vi "ROI_boxes.vi"(11 "Camera Setup":T1={"Analog Gain (0-5)"=4, "Exposure Time"=0.01, "EM Gain (0-255)"=0, "Trigger Polarity"="ATP P", "External Trigger Mode"="ATP P", "Scan Speed"="EMD E", "External Trigger Source"="SSP H", "Scan Mode"="ESC B", "Super Pixel Binning\n(if enabled in Scan Mode)"="SMD N", "Camera Sub-array acquisition region\n(if enabled in scan mode)"={"Left"=0, "Top"=0, "Width"=0, "Height"=0}, "Use camera?"=FALSE, "# image buffers"=100, "shots per measurement"=100, "Force images to U16"=FALSE, "Low Light Sensitivity"="LLS 0", "cooling"="LLS 0", "fan"="LLS 0", "Frame Grabber acquisition region"={"Left"=0, "Top"=0, "Right"=0, "Bottom"=0}} {"Frame Grabber acquisition region"."Bottom" max=512 step=1; "Frame Grabber acquisition region"."Right" max=512 step=1; "Frame Grabber acquisition region"."Top" max=512 step=1; "Frame Grabber acquisition region"."Left" max=512 step=1; "shots per measurement" min=0 step=1; "# image buffers" min=0 step=1; "Camera Sub-array acquisition region\n(if enabled in scan mode)"."Height" min=16 max=512 step=16; "Camera Sub-array acquisition region\n(if enabled in scan mode)"."Width" min=16 max=512 step=16; "Camera Sub-array acquisition region\n(if enabled in scan mode)"."Top" max=496 step=16; "Camera Sub-array acquisition region\n(if enabled in scan mode)"."Left" max=496 step=16; "Analog Gain (0-5)" max=5 step=1}) -> (3 "ROI":T2)   [LabVIEW 2013]
uses:
  Camera/Hamamatsu_C9100-13/camera_setup.ctl
  Camera/Hamamatsu_C9100-13/Hamamatsu_C9100-13.lvclass
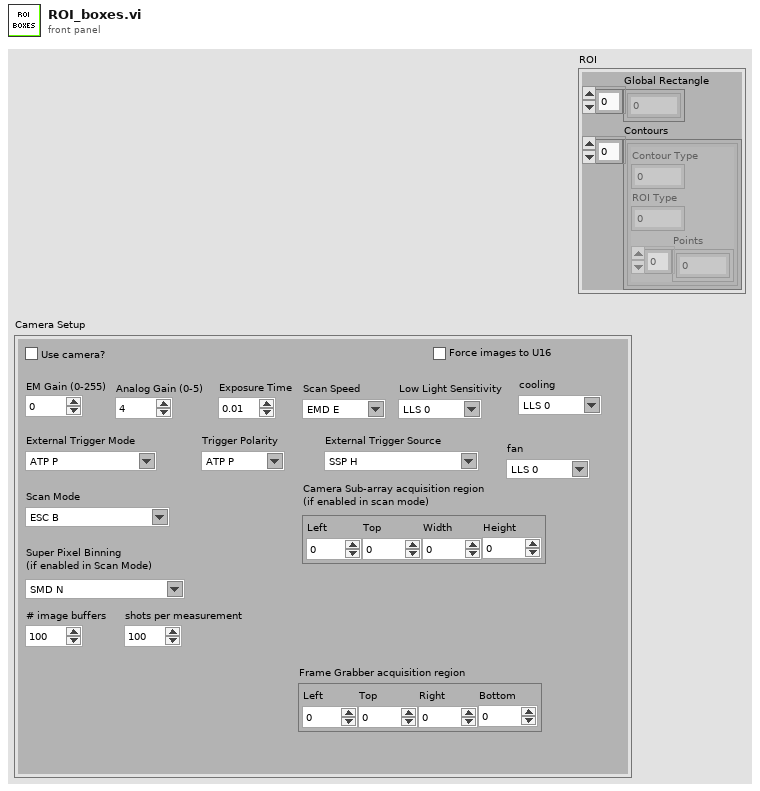
[diagram p1: front panel]
types:
  T1 = typedef "Hamamatsu_C9100-13.lvclass/camera_setup.ctl" = cluster{"Analog Gain (0-5)":u8, "Exposure Time":dbl, "EM Gain (0-255)":u8, "Trigger Polarity":string, "External Trigger Mode":string, "Scan Speed":string, "External Trigger Source":string, "Scan Mode":string, "Super Pixel Binning\n(if enabled in Scan Mode)":string, "Camera Sub-array acquisition region\n(if enabled in scan mode)":cluster{"Left":u16, "Top":u16, "Width":u16, "Height":u16}, "Use camera?":bool, "# image buffers":i32, "shots per measurement":i32, "Force images to U16":bool, "Low Light Sensitivity":string, "cooling":string, "fan":string, "Frame Grabber acquisition region":cluster{"Left":i32, "Top":i32, "Right":i32, "Bottom":i32}}
  T2 = cluster{"Global Rectangle":i32[], "Contours":cluster{"Contour Type":u32, "ROI Type":u32, "Points":i32[]}[]}
  T3 = cluster{"Contour Type":u32, "ROI Type":i32, "Points":i32[]}
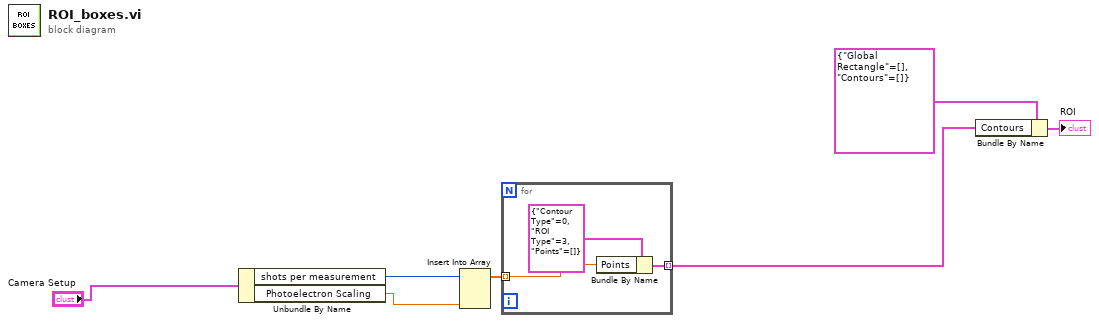
[diagram p0: block diagram]
diagram:
  n1 = Unbundle By Name("Camera Setup") -> ("shots per measurement"=w7:i32, "Photoelectron Scaling"=w6:dbl)
  n2 = Insert Into Array(array=w7, new element=w6) -> (w5:dbl[])  [unwired: 2 in]
  n3 = for {
    tunnel: w5 -> [w9] mode=indexing
    tunnel: [w8] -> w4 mode=indexing
    n4 = Bundle By Name(cluster=T3 {"Contour Type"=0, "ROI Type"=3, "Points"=[]}, "Points"=w9) -> (w8:T3)
  }
  n5 = Bundle By Name(cluster=T2 {"Global Rectangle"=[], "Contours"=[]} ("ROI 2"), "Contours"=w4) -> (→"ROI":T2)
